vi "hatchGrabPiston.vi"(10 "Enum":T1) -> ()   [LabVIEW 2018]
uses:
  HatchGrabPistonEnum.ctl
  <vilib>/Rock Robotics/WPI/Solenoid/WPI_SolenoidValue.ctl
  <vilib>/Rock Robotics/WPI/Solenoid/WPI_SolenoidSetEnum.vi
  <userlib>/836-Library/System/TDMS_V2/Support/Logging_Settings.ctl
  <userlib>/836-Library/System/TDMS_V2/Support/Group_FIFO_Config.ctl
  <userlib>/836-Library/System/TDMS_V2/Support/Channel_FIFO_Config.ctl
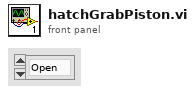
[diagram p1: front panel]
types:
  T1 = typedef "HatchGrabPistonEnum.ctl" = enum16{"Open", "Close"}
  T2 = typedef "Logging_Settings.ctl" = cluster{"Data Grab Period":dbl, "File Write Period":dbl, "Max Stored Size":dbl, "Burst Size":dbl}
  T3 = typedef "Group_FIFO_Config.ctl" = cluster{"Group":string, "Channels":T4[], "Channel Names":string[]}
  T4 = typedef "Channel_FIFO_Config.ctl" = cluster{"Channel":string, "FIFO":refnum<k33>}
  T5 = typedef "Semaphore RefNum" = refnum<k1>
  T6 = cluster{"Name":string, "File Ref":refnum<k34>, "Start Time":timestamp, "Logging Settings":T2, "Group FIFO Config":T3[], "Data To Write":refnum<data-value>, "semaphore":T5, "Ref Time Reset":refnum<k4>}
  T7 = typedef "WPI_SolenoidValue.ctl" = enum16{"Off", "On", "Forward", "Reverse"}
  T8 = typedef "WPI_SolenoidDevRef.ctl" = cluster{"DevStatus":errorcluster, "Pneumatics Control Module":u8, "Forward Solenoid Channel":T9, "Reverse Solenoid Channel":T9}
  T9 = typedef "WPI_SolenoidChannel.ctl" = enum8{"Solenoid 0", "Solenoid 1", "Solenoid 2", "Solenoid 3", "Solenoid 4", "Solenoid 5", "Solenoid 6", "Solenoid 7", "Invalid"}
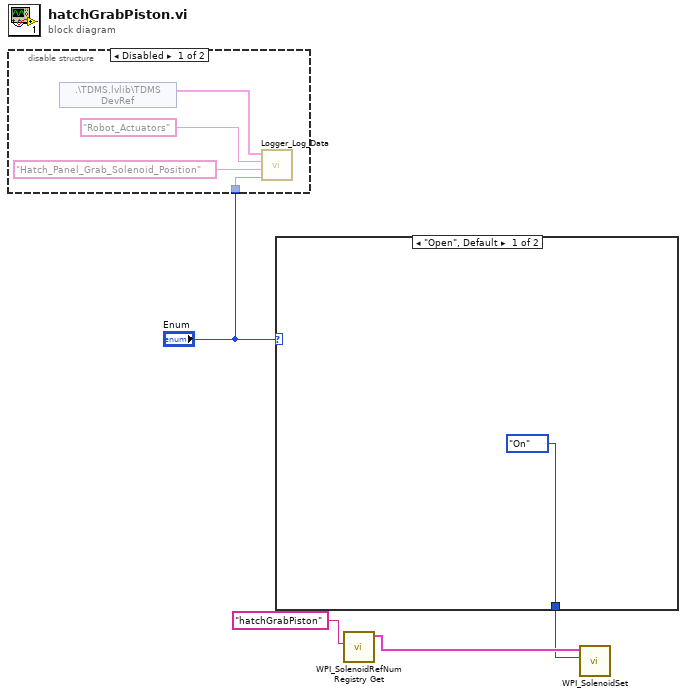
[diagram p0: block diagram]
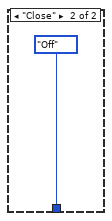
[diagram p3: hidden frame]
diagram:
  n1 = disable-structure shown="Disabled" {
    disable-tunnel: "Enum" -> [w5 _]
    frame Disabled {
      n2 = shared-variable ".\\TDMS.lvlib\\TDMS DevRef"() -> (w7:T6)  [unwired: 1 in, 1 out]
      n3 = call <userlib>:"Logger_Log_Data.vi"("Data"=w5, "Channel"="Hatch_Panel_Grab_Solenoid_Position", "Group"="Robot_Actuators", "TDMS DevRef"=w7) -> ()  [unwired: 7 in, 1 out]
    }
    frame Enabled {
    }
  }
  n4 = case shown="\"Open\", Default" "Enum" {
    tunnel: [WPI_SolenoidValue."On" ("Value") WPI_SolenoidValue."Off" ("Value")] -> w2
    frame "Open", Default {
    }
    frame "Close" {
    }
  }
  n5 = call <vilib>:"WPI_SolenoidRefNum Registry Get.vi"("refnum name"="hatchGrabPiston") -> ("SolenoidDevRef"=w3:T8)  [unwired: 9 in, 1 out]
  n6 = call-poly <vilib>:"WPI_SolenoidSet.vi"("Value"=w2, "SolenoidDevRef"=w3) -> ()  [unwired: 8 in, 2 out]
